vi "FRAS Construction tab XY.vi"(7 "Largeur cote":i32) -> (6 "Tableau X":i32[](array[numeric]), 10 "Tableau Y":i32[](array[numeric]))   [LabVIEW 2020]
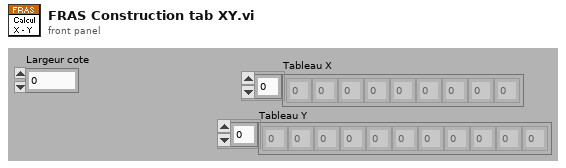
[diagram p1: front panel]
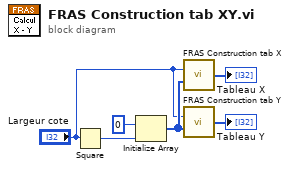
[diagram p0: block diagram]
diagram:
  n1 = Square(x="Largeur cote") -> (x^2=w3:i32)
  n2 = Initialize Array ("Initialiser un tableau")(0 ("élément"), w3) -> (w6:i32[])
  n3 = call "FRAS Construction tab X.vi"("Largeur cote"="Largeur cote", "Tableau"=w6) -> ("Tableau 2"=→"Tableau X":i32[])  [unwired: 13 out]
  n4 = call "FRAS Construction tab Y.vi"("Largeur cote"="Largeur cote", "Tableau"=w6) -> ("Tableau 2"=→"Tableau Y":i32[])  [unwired: 13 out]
